vi "Create FIFO Instance.vi"(7 "Configuration Entry":string, 8 "error in (no error)":errorcluster, 11 "Configuration Parameters":string[](array[string])) -> (0 "error out":errorcluster, 2 "Logic Entry":T1, 3 "Configuration Entry":T1)   [LabVIEW 2021, in "Python Orchestration.lvlib"]
uses:
  Python Orchestration.lvlib
  Typedef/Scripted Line.ctl
  CIFCore/Common/Typedef/Errors.ctl
  <vilib>/CIF Foundation/CIF Utilities/Errors/Append Error Location.vi
  CIFCore/Common/CIFCoreCommon.lvlib
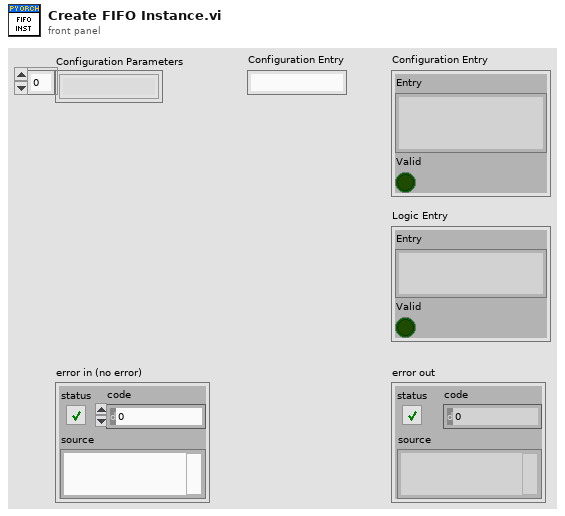
[diagram p1: front panel]
types:
  T1 = typedef "Python Orchestration.lvlib/Scripted Line.ctl" = cluster{"Entry":string, "Valid":bool}
  T2 = typedef "CIFCoreCommon.lvlib/Errors.ctl" = enum16{"Invalid Clock ID", "Long Sleep", "gRPC Server Not Found", "Config Parse", "Timestamp Wrap", "Delayed Execution", "Duplicate Channel", "Missing Channel", "Incorrect Type", "Flatten Error", "Unflatten Data", "Unique Name", "Plugin Not Found", "Plugin Type Not Found", "Plugin Version Not Found", "Manager Not Found", "Numerical Issue", "Time Jump", "Clock ID Match", "Channel Length", "Plugin Connection", "gRPC Server Connection", "PPL Name Match", "Build", "Config Log Parse", "Plugin Load", "UI Subpanel Load", "Python Name", "Invalid Name"}
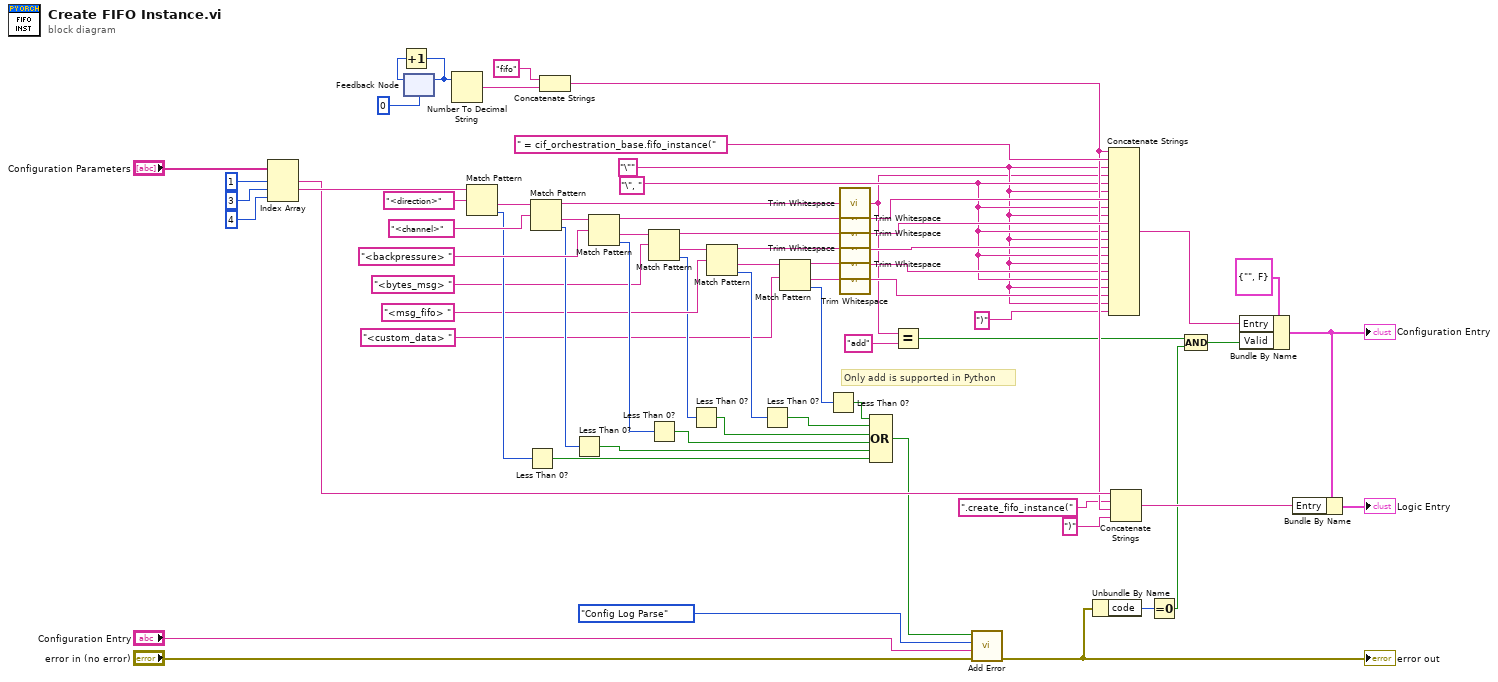
[diagram p0: block diagram]
diagram:
  w20 = "\", "
  w14 = "\""
  # "Only add is supported in Python"
  n1 = Index Array(array="Configuration Parameters", index #1=1 ("index"), index #2=3 ("index"), index #3=4 ("index")) -> (element #1=w38:string, element #2=w54:string)  [unwired: 1 out]
  n2 = feedback #1(u16 0) -> (w58:u16)
  n3 = Increment(x=w58) -> (x+1=w57:u16)
  n4 = feedback-in #1(w57) -> ()
  n5 = Number To Decimal String(number=w57) -> (decimal integer string=w55:string)  [unwired: 1 in]
  n6 = Match Pattern(string=w54, regular expression="<direction>") -> (after substring=w61:string, offset past match=w42:i32)  [unwired: 1 in, 2 out]
  n7 = Less Than 0?(x=w42) -> (x < 0?=w41:bool)
  n8 = Match Pattern(string=w61, regular expression="<channel>") -> (before substring=w52:string, after substring=w51:string, offset past match=w43:i32)  [unwired: 1 in, 1 out]
  n9 = Concatenate Strings("fifo" ("string"), w55) -> (w37:string)
  n10 = Less Than 0?(x=w43) -> (x < 0?=w40:bool)
  n11 = Match Pattern(string=w51, regular expression="<backpressure> ") -> (before substring=w49:string, after substring=w35:string, offset past match=w44:i32)  [unwired: 1 in, 1 out]
  n12 = Match Pattern(string=w35, regular expression="<bytes_msg> ") -> (before substring=w27:string, after substring=w33:string, offset past match=w31:i32)  [unwired: 1 in, 1 out]
  n13 = Less Than 0?(x=w44) -> (x < 0?=w39:bool)
  n14 = Less Than 0?(x=w31) -> (x < 0?=w30:bool)
  n15 = Match Pattern(string=w33, regular expression="<msg_fifo> ") -> (before substring=w26:string, after substring=w23:string, offset past match=w29:i32)  [unwired: 1 in, 1 out]
  n16 = Less Than 0?(x=w29) -> (x < 0?=w28:bool)
  n17 = Match Pattern(string=w23, regular expression="<custom_data> ") -> (before substring=w22:string, after substring=w21:string, offset past match=w18:i32)  [unwired: 1 in, 1 out]
  n18 = Less Than 0?(x=w18) -> (x < 0?=w17:bool)
  n19 = call <vilib>:"Trim Whitespace.vi"("string"=w52) -> ("trimmed string"=w12:string)  [unwired: 1 in]
  n20 = call <vilib>:"Trim Whitespace.vi"("string"=w49) -> ("trimmed string"=w48:string)  [unwired: 1 in]
  n21 = call <vilib>:"Trim Whitespace.vi"("string"=w27) -> ("trimmed string"=w47:string)  [unwired: 1 in]
  n22 = call <vilib>:"Trim Whitespace.vi"("string"=w26) -> ("trimmed string"=w25:string)  [unwired: 1 in]
  n23 = call <vilib>:"Trim Whitespace.vi"("string"=w22) -> ("trimmed string"=w24:string)  [unwired: 1 in]
  n24 = call <vilib>:"Trim Whitespace.vi"("string"=w21) -> ("trimmed string"=w19:string)  [unwired: 1 in]
  n25 = Compound Arithmetic op=OR(w17, w28, w30, w39, w40, w41) -> (w1:bool)
  n26 = Equal?(x=w12, y="add") -> (x = y?=w10:bool)
  n27 = call "Add Error.vi"("error in (no error)"="error in (no error)", "String to Append"="Configuration Entry", "Error"=Errors."Config Log Parse", "Insert Error"=w1) -> ("error out"=w4:errorcluster)  [unwired: 7 in]
  "error out" <- w4
  n28 = Unbundle By Name(w4) -> ("code"=w68:i32)
  n29 = Concatenate Strings(w37, " = cif_orchestration_base.fifo_instance(", w14, w12, w20, w14, w48, w20, w14, w47, w20, w14, w25, w20, w14, w24, w20, w14, w19, w14, ")" ("string")) -> (w46:string)
  n30 = Concatenate Strings(w38, ".create_fifo_instance(" ("string"), w37, ")" ("string")) -> (w45:string)
  n31 = Equal To 0?(x=w68) -> (x = 0?=w9:bool)
  n32 = Compound Arithmetic op=AND(w10, w9) -> (w8:bool)
  n33 = Bundle By Name(cluster=T1 {"Entry"="", "Valid"=FALSE} ("Logic Entry"), "Entry"=w46, "Valid"=w8) -> (w36:T1)
  "Configuration Entry" <- w36
  n34 = Bundle By Name(cluster=w36, "Entry"=w45) -> (→"Logic Entry":T1)
